vi "DMM Switch Handshaking - Cycle Time.vi"(8 "error in":errorcluster, 11 "file path (use dialog)":path=path "C:/OCVtestfile.json") -> (0 "error out":errorcluster, 2 "Results":T1={"V ch0 Array"=[2.6402355104591723e-06, 3.2050422226470716e-06, 3.2738385547093894e-06, 3.0004056082675545e-06, 3.190429018678622e-06, 3.265655292871135e-06, 3.4283206777974678e-06], "V ch1 Array"=[3.579181433209794e-06, 3.538102305000126e-06, 3.3674070559982216e-06, 3.2951997357567907e-06, 3.0614196043446336e-06, 3.247982674682344e-06, 3.4582756481500834e-06], "V ch2 Array"=[2.636942617106564e-06, 2.444215695573972e-06, 2.3600385872845126e-06, 2.3785120159418297e-06, 2.39158079459529e-06, 2.5415574149365358e-06, 2.629696833600491e-06], "V ch3 Array"=[4.29015971742814e-06, 4.582682915243894e-06, 4.199947801068903e-06, 4.210565880465411e-06, 4.1249236933492e-06, 4.3283146693326225e-06], "V ch4 Array"=[3.2068632920738282e-06, 3.2352868353418705e-06, 3.218523090660476e-06, 3.1985005992771743e-06, 3.2252632419667723e-06, 3.3472279144313767e-06], "Elapsed Time (ms)"=11164, "DMM Fault Array"=[]})   [LabVIEW 2019]
uses:
  OCVResults.ctl
  OCVJSONCluster.ctl
  <instrlib>/niDMM/nidmm.llb/niDMM Configure Measurement Digits.vi
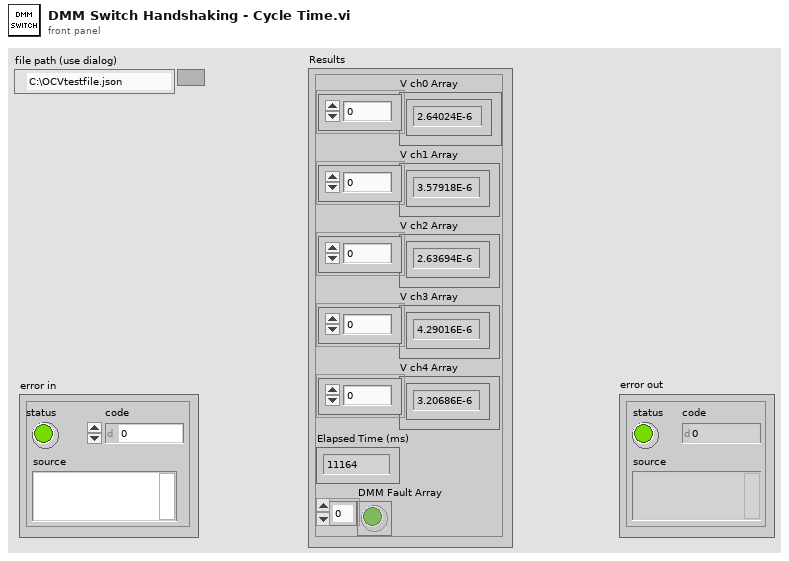
[diagram p1: front panel]
types:
  T1 = typedef "OCVResults.ctl" = cluster{"V ch0 Array":dbl[], "V ch1 Array":dbl[], "V ch2 Array":dbl[], "V ch3 Array":dbl[], "V ch4 Array":dbl[], "Elapsed Time (ms)":u32, "DMM Fault Array":bool[]}
  T2 = typedef "OCVJSONCluster.ctl" = cluster{"SwitchResourceName":string, "SwitchTopology":string, "SwitchInputTrigger_TTL0":i32, "SwitchScanAdvancedOutput_TTL1":i32, "SwitchScanList":string, "DMMResourceName":string, "DMMFunction_DCVolts":i32, "DMMResolution":dbl, "DMMRange":dbl, "DMMTriggerSource_TTL1":i32, "DMMTriggerSlope_RisingEdge":i32, "DMMSampleTrigger_TTL1":i32, "DMMSampleCount":i32, "DMMSampleTriggerSlope_RisingEdge":i32, "DMMMeasurementCompleteTrigger_TTL0":i32, "DMMMeasurementCompleteTriggerSlope_RisingEdge":i32, "DMMApertureTimeUnits_Seconds":i32, "DMMApertureTime":dbl, "DMMNumberOfAverages":i32, "DMMAutoZero_Off":i32, "DMMADCCalibration_Off":i32, "DMMSettleTime":dbl, "DMMControlAction_Commit":i32, "ApplicationLoopCount":i32, "ApplicationNumberOfBatteryCells":i32}
  T3 = enum16{"open", "replace", "create", "open or create", "replace or create", "replace or create with confirmation"}
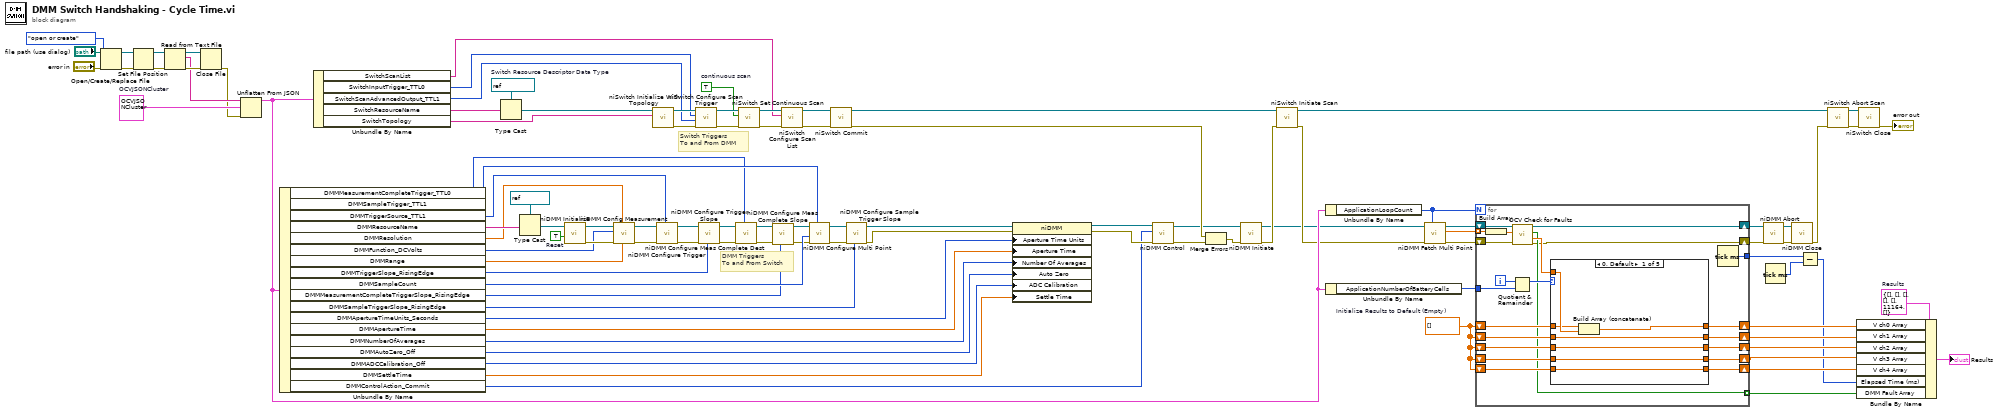
[diagram p0: block diagram]
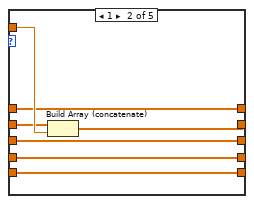
[diagram p2: hidden frame]
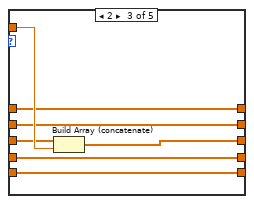
[diagram p3: hidden frame]
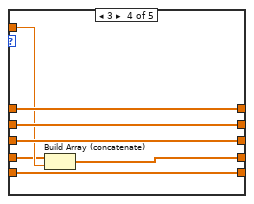
[diagram p4: hidden frame]
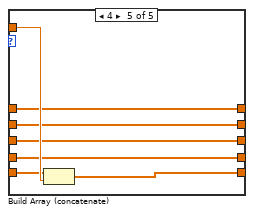
[diagram p5: hidden frame]
diagram:
  w44 = refnum<k15> "Switch"  # Switch Resource Descriptor Data Type
  w66 = T2 {"SwitchResourceName"="", "SwitchTopology"="", "SwitchInputTrigger_TTL0"=0, "SwitchScanAdvancedOutput_TTL1"=0, "SwitchScanList"="", "DMMResourceName"="", "DMMFunction_DCVolts"=0, "DMMResolution"=0.0, "DMMRange"=0.0, "DMMTriggerSource_TTL1"=0, "DMMTriggerSlope_RisingEdge"=0, "DMMSampleTrigger_TTL1"=0, "DMMSampleCount"=0, "DMMSampleTriggerSlope_RisingEdge"=0, "DMMMeasurementCompleteTrigger_TTL0"=0, "DMMMeasurementCompleteTriggerSlope_RisingEdge"=0, "DMMApertureTimeUnits_Seconds"=0, "DMMApertureTime"=0.0, "DMMNumberOfAverages"=0, "DMMAutoZero_Off"=0, "DMMADCCalibration_Off"=0, "DMMSettleTime"=0.0, "DMMControlAction_Commit"=0, "ApplicationLoopCount"=0, "ApplicationNumberOfBatteryCells"=0}  # OCVJSONCluster
  w52 = T1 {"V ch0 Array"=[], "V ch1 Array"=[], "V ch2 Array"=[], "V ch3 Array"=[], "V ch4 Array"=[], "Elapsed Time (ms)"=11164, "DMM Fault Array"=[]}  # Results
  w54 = dbl[] []  # Initialize Results to Default (Empty)
  w86 = TRUE  # Reset
  w99 = TRUE  # continuous scan
  # "Switch Triggers\nTo and From DMM"
  # "DMM Triggers\nTo and From Switch"
  n1 = Open/Create/Replace File(file path (use dialog)="file path (use dialog)", error in="error in", operation (0:open)=T3."open or create") -> (refnum out=w59:refnum<file>, error out=w58:errorcluster)  [unwired: 3 in, 1 out]
  n2 = Set File Position(refnum=w59, error in=w58) -> (refnum out=w61:refnum<file>, error out=w60:errorcluster)  [unwired: 2 in]
  n3 = Read from Text File(file (use dialog)=w61, error in=w60) -> (refnum out=w63:refnum<file>, text=w57:string, error out=w62:errorcluster)  [unwired: 2 in, 1 out]
  n4 = Close File(refnum=w63, error in=w62) -> (error out=w56:errorcluster)  [unwired: 1 out]
  n5 = Unflatten From JSON(JSON string=w57, type and defaults=w66, error in (no error)=w56) -> (value=w29:T2)  [unwired: 4 in, 1 out]
  n6 = Unbundle By Name(w29) -> ("DMMMeasurementCompleteTrigger_TTL0"=w17:i32, "DMMSampleTrigger_TTL1"=w31:i32, "DMMTriggerSource_TTL1"=w37:i32, "DMMResourceName"=w28:string, "DMMResolution"=w27:dbl, "DMMFunction_DCVolts"=w34:i32, "DMMRange"=w36:dbl, "DMMTriggerSlope_RisingEdge"=w35:i32, "DMMSampleCount"=w33:i32, "DMMMeasurementCompleteTriggerSlope_RisingEdge"=w16:i32, "DMMSampleTriggerSlope_RisingEdge"=w32:i32, "DMMApertureTimeUnits_Seconds"=w1:i32, "DMMApertureTime"=w2:dbl, "DMMNumberOfAverages"=w6:i32, "DMMAutoZero_Off"=w3:i32, "DMMADCCalibration_Off"=w5:i32, "DMMSettleTime"=w4:dbl, "DMMControlAction_Commit"=w18:i32)
  n7 = Unbundle By Name(w29) -> ("SwitchScanList"=w7:string, "SwitchInputTrigger_TTL0"=w42:i32, "SwitchScanAdvancedOutput_TTL1"=w15:i32, "SwitchResourceName"=w41:string, "SwitchTopology"=w40:string)
  n8 = Type Cast(type=w44, x=w41) -> (*(type *) &x=w43:refnum<k15>)
  n9 = Type Cast(type=refnum<k15> "DMM" ("Device Name"), x=w28) -> (*(type *) &x=w38:refnum<k15>)
  n10 = call <instrlib>:"niDMM Initialize.vi"("Reset"=w86, "Instrument Descriptor"=w38) -> ("error out"=w77:errorcluster, "instrument handle out"=w76:refnum<k15>)  [unwired: 8 in]
  n11 = call-poly <instrlib>:"niDMM Config Measurement.vi"("Range"=w36, "Resolution in Digits"=w27, "error in (no error)"=w77, "Function"=w34, "instrument handle"=w76) -> ("error out"=w81:errorcluster, "instrument handle out"=w80:refnum<k15>)  [unwired: 5 in]
  n12 = call <instrlib>:"niSwitch Initialize With Topology.vi"("topology name"=w40, "resource name"=w43) -> ("error out"=w96:errorcluster, "instrument handle out"=w97:refnum<k15>)  [unwired: 3 in, 5 out]
  n13 = call <instrlib>:"niDMM Configure Trigger.vi"("Trigger Source"=w37, "error in (no error)"=w81, "instrument handle"=w80) -> ("error out"=w83:errorcluster, "instrument handle out"=w82:refnum<k15>)  [unwired: 7 in]
  n14 = call <instrlib>:"niSwitch Configure Scan Trigger.vi"("error in (no error)"=w96, "scan advanced output (External)"=w15, "trigger input (External)"=w42, "instrument handle"=w97) -> ("error out"=w100:errorcluster, "instrument handle out"=w102:refnum<k15>)  [unwired: 1 in, 5 out]
  n15 = call <instrlib>:"niDMM Configure Trigger Slope.vi"("Slope"=w35, "error in (no error)"=w83, "instrument handle"=w82) -> ("error out"=w23:errorcluster, "instrument handle out"=w24:refnum<k15>)  [unwired: 7 in]
  n16 = call <instrlib>:"niDMM Configure Meas Complete Dest.vi"("Measurement Complete Destination"=w17, "error in (no error)"=w23, "instrument handle"=w24) -> ("error out"=w21:errorcluster, "instrument handle out"=w22:refnum<k15>)  [unwired: 7 in]
  n17 = call <instrlib>:"niSwitch Set Continuous Scan.vi"("error in (no error)"=w100, "continuous scan (False)"=w99, "instrument handle"=w102) -> ("error out"=w94:errorcluster, "instrument handle out"=w95:refnum<k15>)  [unwired: 7 out]
  n18 = call <instrlib>:"niDMM Configure Meas Complete Slope.vi"("Slope"=w16, "error in (no error)"=w21, "instrument handle"=w22) -> ("error out"=w20:errorcluster, "instrument handle out"=w19:refnum<k15>)  [unwired: 7 in]
  n19 = call <instrlib>:"niSwitch Configure Scan List.vi"("error in (no error)"=w94, "scan list"=w7, "instrument handle"=w95) -> ("error out"=w92:errorcluster, "instrument handle out"=w91:refnum<k15>)  [unwired: 1 in, 6 out]
  n20 = call <instrlib>:"niDMM Configure Multi Point.vi"("Sample Trigger"=w31, "error in (no error)"=w20, "Sample Count"=w33, "instrument handle"=w19) -> ("error out"=w85:errorcluster, "instrument handle out"=w84:refnum<k15>)  [unwired: 6 in]
  n21 = call <instrlib>:"niSwitch Commit.vi"("error in (no error)"=w92, "instrument handle"=w91) -> ("error out"=w75:errorcluster, "instrument handle out"=w90:refnum<k15>)  [unwired: 8 out]
  n22 = call <instrlib>:"niDMM Configure Sample Trigger Slope.vi"("Slope"=w32, "error in (no error)"=w85, "instrument handle"=w84) -> ("error out"=w70:errorcluster, "instrument handle out"=w71:refnum<k15>)  [unwired: 7 in]
  n23 = property class="niDMM"(reference=w71, error in=w70, "Aperture Time Units"=w1, "Aperture Time"=w2, "Number Of Averages"=w6, "Auto Zero"=w3, "ADC Calibration"=w5, "Settle Time"=w4) -> (reference out=w68:refnum<k15>, error out=w67:errorcluster)
  n24 = call <instrlib>:"niDMM Control.vi"("error in (no error)"=w67, "Control Action"=w18, "instrument handle"=w68) -> ("error out"=w74:errorcluster, "instrument handle out"=w72:refnum<k15>)  [unwired: 7 in]
  n25 = Merge Errors(w75, w74) -> (w73:errorcluster)
  n26 = call <instrlib>:"niDMM Initiate.vi"("error in (no error)"=w73, "instrument handle"=w72) -> ("error out"=w26:errorcluster, "instrument handle out"=w13:refnum<k15>)  [unwired: 8 in]
  n27 = call <instrlib>:"niSwitch Initiate Scan.vi"("error in (no error)"=w26, "instrument handle"=w90) -> ("error out"=w14:errorcluster, "instrument handle out"=w93:refnum<k15>)  [unwired: 8 out]
  n28 = Unbundle By Name(w29) -> ("ApplicationLoopCount"=w11:i32)
  n29 = Unbundle By Name(w29) -> ("ApplicationNumberOfBatteryCells"=w30:i32)
  n30 = call <instrlib>:"niDMM Fetch Multi Point.vi"("Number to Fetch"=w11, "error in (no error)"=w14, "instrument handle"=w13) -> ("error out"=w10:errorcluster, "Measurements"=w12:dbl[], "instrument handle out"=w9:refnum<k15>)  [unwired: 5 in, 1 out]
  n31 = for {
    N: w11 -> [_]
    shift-right: [w107] -> w69
    shift-left: w10 -> [w106]
    tunnel: [w123] -> w88
    shift-right: [w103] -> w8
    shift-left: w9 -> [w103]
    shift-right: [w120] -> w53
    shift-left: w54 -> [w119]
    shift-right: [w118] -> w48
    shift-left: w54 -> [w117]
    shift-right: [w116] -> w49
    shift-left: w54 -> [w115]
    shift-right: [w114] -> w50
    shift-left: w54 -> [w113]
    shift-right: [w112] -> w51
    shift-left: w54 -> [w111]
    tunnel: [w109] -> w45 mode=indexing
    tunnel: w30 -> [w108]
    tunnel: w12 -> [w105] mode=indexing
    i -> [w122]
    n32 = Build Array(w105) -> (w104:dbl[])
    n33 = call "OCV Check for Faults.vi"("Error In"=w106, "dmm voltage measurements"=w104) -> ("Error Out"=w107:errorcluster, "Voltage Out"=w110:dbl, "DMM Fault"=w109:bool)  [unwired: 7 in]
    n34 = Quotient & Remainder(x=w122, y=w108) -> (x-y*floor(x/y)=w121:i32)  [unwired: 1 out]
    n35 = case shown="0, Default" w121 {
      tunnel: w110 -> [w130 w137 w144 w148 w158]
      tunnel: [w129 w134 w141 w151 w155] -> w120
      tunnel: w119 -> [w128 w134 w141 w151 w155]
      tunnel: [w127 w136 w140 w150 w154] -> w118
      tunnel: w117 -> [w127 w135 w140 w150 w154]
      tunnel: [w126 w133 w143 w149 w153] -> w116
      tunnel: w115 -> [w126 w133 w142 w149 w153]
      tunnel: [w125 w132 w139 w147 w152] -> w114
      tunnel: w113 -> [w125 w132 w139 w146 w152]
      tunnel: [w124 w131 w138 w145 w157] -> w112
      tunnel: w111 -> [w124 w131 w138 w145 w156]
      frame 0, Default {
        n36 = Build Array (concatenate)(w128, w130) -> (w129:dbl[])
      }
      frame 1 {
        n37 = Build Array (concatenate)(w135, w137) -> (w136:dbl[])
      }
      frame 2 {
        n38 = Build Array (concatenate)(w142, w144) -> (w143:dbl[])
      }
      frame 3 {
        n39 = Build Array (concatenate)(w146, w148) -> (w147:dbl[])
      }
      frame 4 {
        n40 = Build Array (concatenate)(w156, w158) -> (w157:dbl[])
      }
    }
    n41 = Tick Count (ms)() -> (millisecond timer value=w123:u32)
  }
  n42 = call <instrlib>:"niDMM Abort.vi"("error in (no error)"=w69, "instrument handle"=w8) -> ("error out"=w79:errorcluster, "instrument handle out"=w78:refnum<k15>)  [unwired: 8 in]
  n43 = Tick Count (ms)() -> (millisecond timer value=w87:u32)
  n44 = call <instrlib>:"niDMM Close.vi"("error in (no error)"=w79, "instrument handle"=w78) -> ("error out"=w25:errorcluster)  [unwired: 9 in]
  n45 = Subtract(x=w88, y=w87) -> (x-y=w46:u32)
  n46 = call <instrlib>:"niSwitch Abort Scan.vi"("error in (no error)"=w25, "instrument handle"=w93) -> ("error out"=w98:errorcluster, "instrument handle out"=w101:refnum<k15>)  [unwired: 8 out]
  n47 = Bundle By Name(cluster=w52, "V ch0 Array"=w53, "V ch1 Array"=w48, "V ch2 Array"=w49, "V ch3 Array"=w50, "V ch4 Array"=w51, "Elapsed Time (ms)"=w46, "DMM Fault Array"=w45) -> (→"Results":T1)
  n48 = call <instrlib>:"niSwitch Close.vi"("error in (no error)"=w98, "instrument handle"=w101) -> ("error out"=→"error out":errorcluster)  [unwired: 9 out]
